vi "Ballard - Arinc-429 - Main Page.vi"(8 "error in (no error)":errorcluster, 11 "Node Ptr":T1 format="%.0x") -> (0 "error out":errorcluster)   [LabVIEW 2016, in "Ballard Arinc-429 System Explorer.lvlib"]
uses:
  Ballard Arinc-429 System Explorer.lvlib
  <vilib>/NI Veristand/Custom Device API/Custom Device Item Ref.ctl
  Shared/Controls and Global/Global.vi
  <vilib>/NI Veristand/Custom Device API/Get Item Property (Boolean).vi
  <vilib>/NI Veristand/Custom Device API/Get Item Property (Path).vi
  <vilib>/NI Veristand/Custom Device API/Get Item Property (String).vi
  <vilib>/NI Veristand/Custom Device API/Get Item Property (I32).vi
  <vilib>/NI Veristand/Custom Device API/Set Item Property (I32).vi
  <vilib>/NI Veristand/Custom Device API/Set Item Property (String).vi
  <vilib>/NI Veristand/Custom Device API/Custom Device API.lvlib
  Shared/Ballard Arinc-429 Shared.lvlib
  <vilib>/NI Veristand/Custom Device API/Set Item Property (Boolean).vi
panel:
  in  "Core Number":i32
  in  "Card Number":i32
  out "Version":string
  in  "ScheduledSDI?":bool
  in  "RefreshDB":bool
  in  "Warning text":string="WARNING: The database has changed since import. If you attempt to run this system definition an error may occur. Consider refreshing the database import."
  out "Warn Icon":bool
  out "Database File":path
  in  "Header":cluster{"Section Name":string}={"Section Name"="Ballard - Arinc-429 -  Custom Device"}
  in  "Description":string
  in  "Name":string
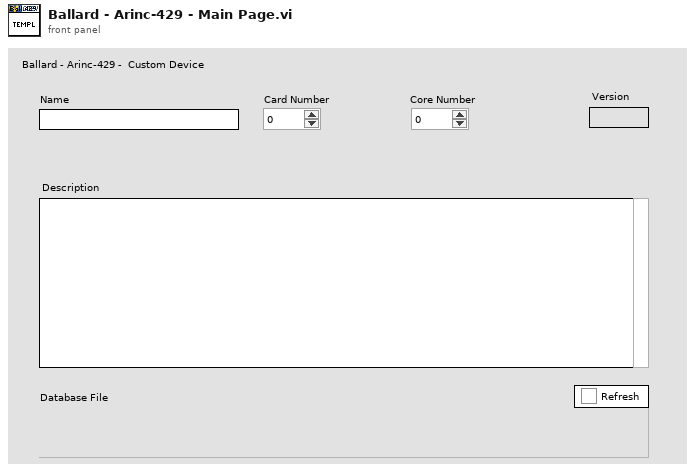
[diagram p1: front panel]
types:
  T1 = typedef "Custom Device API.lvlib/Custom Device Item Ref.ctl" = u64
  T2 = typedef "Custom Device API.lvlib/Custom Device Item Info.ctl" = cluster{"Name":string, "Is Channel":bool, "GUID":string, "Is Waveform":bool}
  T3 = typedef "Custom Device API.lvlib/Custom Device Commands.ctl" = enum16{"Default", "Item renamed", "Shutdown", "Dynamic button pressed"}
  T4 = typedef "Ballard Arinc-429 System Explorer.lvlib/Refresh Match Settings.ctl" = cluster{"Ch by name?":bool, "Lbl by name?":bool}
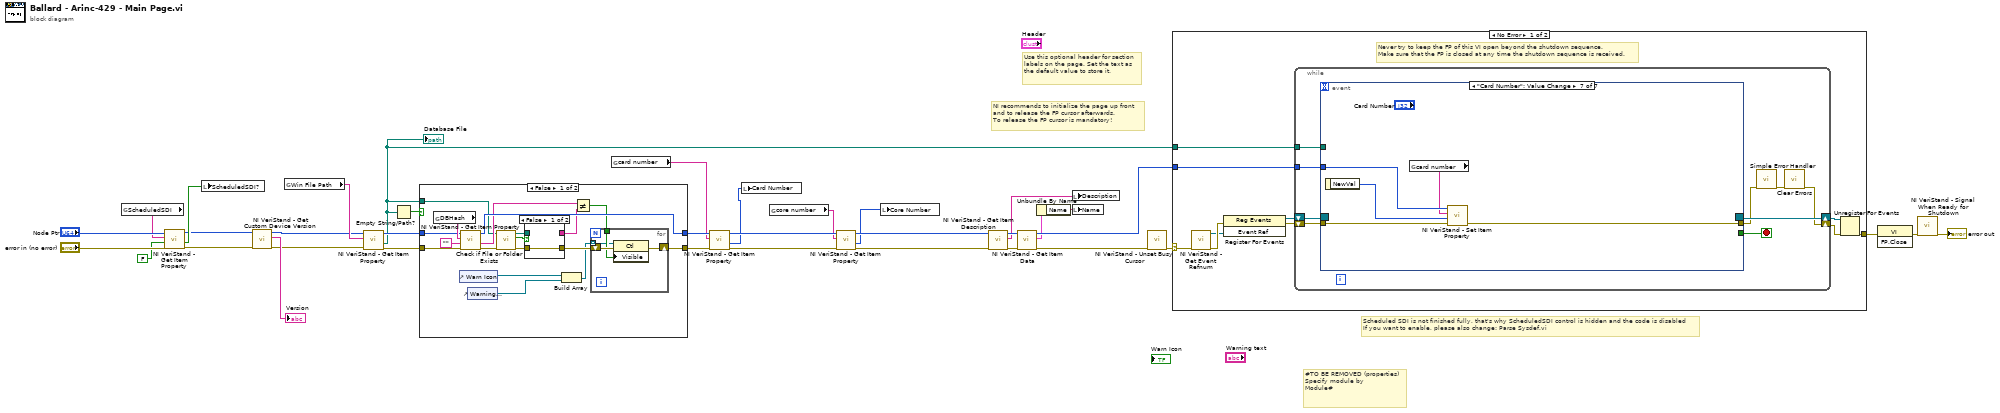
[diagram p0: block diagram]
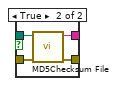
[diagram p2: hidden frame]
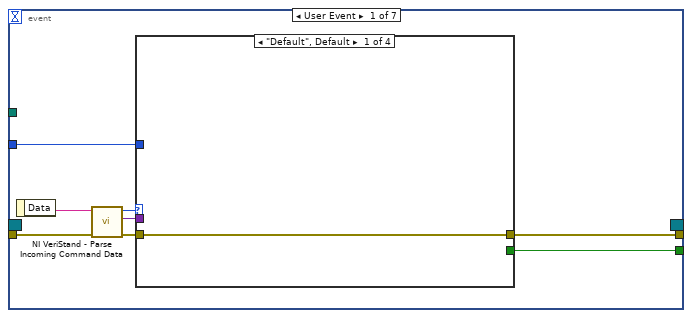
[diagram p4: hidden frame]
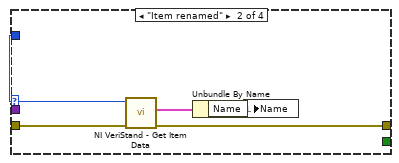
[diagram p5: hidden frame]
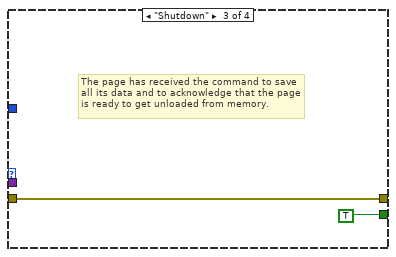
[diagram p6: hidden frame]
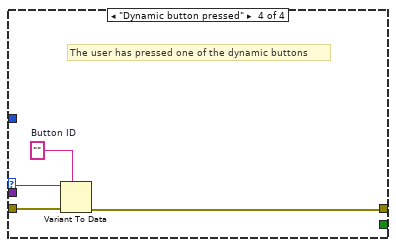
[diagram p7: hidden frame]
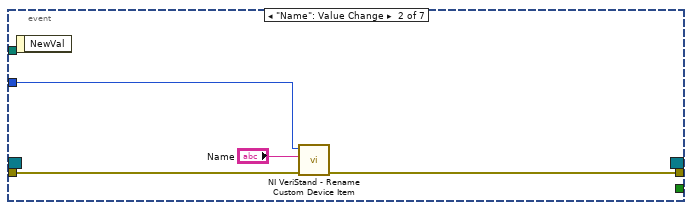
[diagram p8: hidden frame]
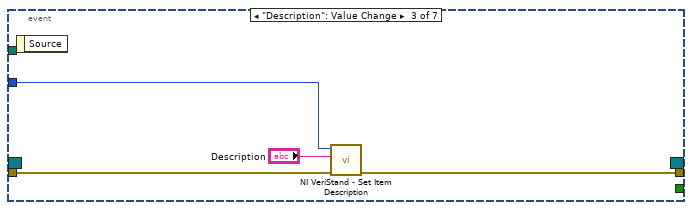
[diagram p9: hidden frame]
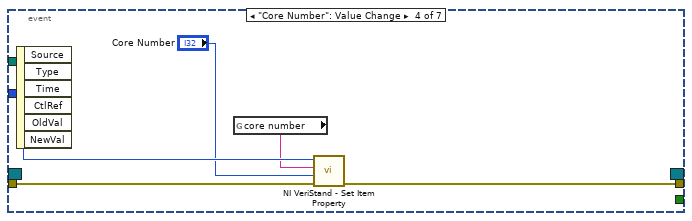
[diagram p10: hidden frame]
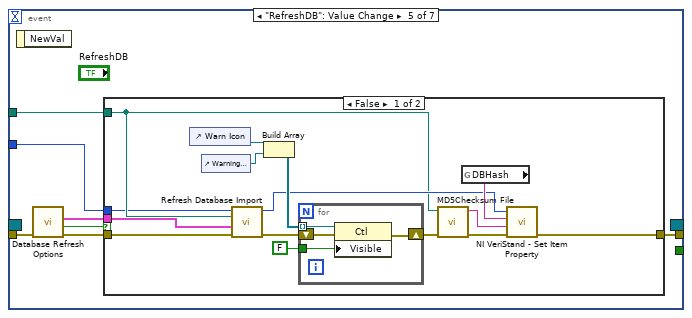
[diagram p11: hidden frame]
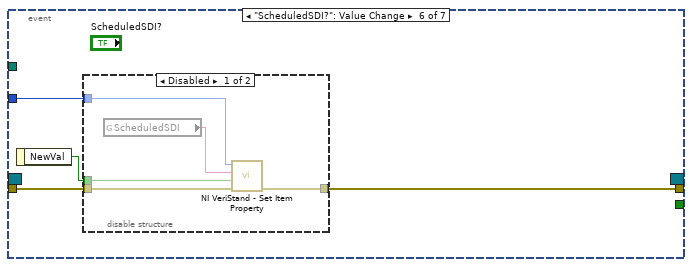
[diagram p13: hidden frame]
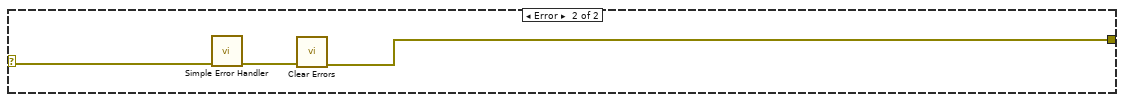
[diagram p15: hidden frame]
diagram:
  # "#TO BE REMOVED (properties)\nSpecify module by\nModule#"
  # "Scheduled SDI is not finished fully, that's why ScheduledSDI control is hidden and the code is disabled\nIf you want to enable, please also change: Parse Sysdef.vi"
  # "Use this optional header for section labels on the page. Set the text as the default value to store it."
  # "NI recommends to initialize the page up front\nand to release the FP cursor afterwards.\nTo release the FP cursor is mandatory!"
  n1 = global read "Global.vi" "ScheduledSDI"() -> (w15:string)
  n2 = call-poly <vilib>:"NI VeriStand - Get Item Property.vi"("error in (no error)"="error in (no error)", "Default Value"=FALSE, "Property Name"=w15, "Item Ref in"="Node Ptr") -> ("error out"=w16:errorcluster, "Value"=w13:bool, "Item Ref out"=w12:T1)  [unwired: 4 in, 1 out]
  n3 = local write "ScheduledSDI?"(w13) -> ()
  n4 = call <vilib>:"NI VeriStand - Get Custom Device Version.vi"("error in (no error)"=w16, "Device Ref in"=w12) -> ("error out"=w9:errorcluster, "Value"=→"Version":string, "Device Ref out"=w10:T1)  [unwired: 7 in]
  n5 = global read "Global.vi" "Win File Path"() -> (w25:string)
  n6 = call-poly <vilib>:"NI VeriStand - Get Item Property.vi"("error in (no error)"=w9, "Property Name"=w25, "Item Ref in"=w10) -> ("error out"=w23:errorcluster, "Value"=w19:path, "Item Ref out"=w20:T1)  [unwired: 5 in, 1 out]
  "Database File" <- w19
  n7 = Empty String/Path?(string/path=w19) -> (empty?=w24:bool)
  n8 = case shown="False" w24 {
    tunnel: w23 -> [w51 w65]
    tunnel: [w42 w65] -> w22
    tunnel: [w50 w64] -> w21
    tunnel: w20 -> [w52 w64]
    tunnel: w19 -> [w38 _]
    frame False {
      n9 = global read "Global.vi" "DBHash"() -> (w53:string)
      n10 = control-ref of="Warn Icon"() -> (w44:refnum<vi>)
      n11 = call-poly <vilib>:"NI VeriStand - Get Item Property.vi"("error in (no error)"=w51, "Default Value"="", "Property Name"=w53, "Item Ref in"=w52) -> ("error out"=w39:errorcluster, "Value"=w48:string, "Item Ref out"=w50:T1)  [unwired: 4 in, 1 out]
      n12 = control-ref of="Warning text"() -> (w45:refnum<vi>)
      n13 = call <vilib>:"Check if File or Folder Exists.vi"("error in (no error)"=w39, "path"=w38) -> ("error out"=w41:errorcluster, "file or folder exists?"=w37:bool, "dup path"=w40:path)  [unwired: 7 in]
      n14 = case shown="False" w37 {
        tunnel: [_ w59] -> w49
        tunnel: [w55 w58] -> w47
        tunnel: w41 -> [w55 w57]
        tunnel: w40 -> [_ w56]
        frame False {
        }
        frame True {
          n15 = call <vilib>:"MD5Checksum File.vi"("error in (no error)"=w57, "Path"=w56) -> ("error out"=w58:errorcluster, "MD5 message-digest"=w59:string)  [unwired: 8 in]
        }
      }
      n16 = Build Array(w44, w45) -> (w43:refnum<vi>[])
      n17 = Not Equal?(x=w48, y=w49) -> (x != y?=w46:bool)
      n18 = for {
        shift-right: [w62] -> w42
        shift-left: w47 -> [w63]
        tunnel: w46 -> [w61]
        tunnel: w43 -> [w60] mode=indexing
        n19 = property class="Ctl"(reference=w60, error in=w63, "Visible"=w61) -> (error out=w62:errorcluster)  [unwired: 1 out]
      }
    }
    frame True {
    }
  }
  n20 = global read "Global.vi" "card number"() -> (w2:string)
  n21 = call-poly <vilib>:"NI VeriStand - Get Item Property.vi"("error in (no error)"=w22, "Property Name"=w2, "Item Ref in"=w21) -> ("error out"=w5:errorcluster, "Value"=w1:i32, "Item Ref out"=w7:T1)  [unwired: 5 in, 1 out]
  n22 = local write "Card Number"(w1) -> ()
  n23 = global read "Global.vi" "core number"() -> (w3:string)
  n24 = call-poly <vilib>:"NI VeriStand - Get Item Property.vi"("error in (no error)"=w5, "Property Name"=w3, "Item Ref in"=w7) -> ("error out"=w8:errorcluster, "Value"=w4:i32, "Item Ref out"=w6:T1)  [unwired: 5 in, 1 out]
  n25 = local write "Core Number"(w4) -> ()
  n26 = call <vilib>:"NI VeriStand - Get Item Description.vi"("error in (no error)"=w8, "Item Ref in"=w6) -> ("error out"=w28:errorcluster, "Description"=w29:string, "Item Ref out"=w30:T1)  [unwired: 7 out]
  n27 = call <vilib>:"NI VeriStand - Get Item Data.vi"("error in (no error)"=w28, "Item Ref in"=w30) -> ("error out"=w33:errorcluster, "Item Info"=w27:T2, "Item Ref out"=w31:T1)  [unwired: 7 out]
  n28 = Unbundle By Name(w27) -> ("Name"=w26:string)
  n29 = local write "Description"(w29) -> ()
  n30 = local write "Name"(w26) -> ()
  n31 = call <vilib>:"NI VeriStand - Unset Busy Cursor.vi"("error in (no error)"=w33) -> ("error out"=w32:errorcluster)  [unwired: 10 out]
  n32 = case shown="No Error" w32 {
    selector: w32 -> [w67 w162]
    tunnel: [w72 w160] -> w36
    tunnel: w31 -> [w68 _]
    tunnel: w19 -> [w66 _]
    frame No Error {
      # "Never try to keep the FP of this VI open beyond the shutdown sequence.\nMake sure that the FP is closed at any time the shutdown sequence is received."
      n33 = call <vilib>:"NI VeriStand - Get Event Refnum.vi"("error in (no error)"=w67) -> ("error out"=w75:errorcluster, "Event Ref"=w71:refnum<user-event>)  [unwired: 9 out]
      n34 = register-events(error in=w75, w71) -> (reference out=w69:refnum<event-registration>, error out=w70:errorcluster)  [unwired: 1 in]
      n35 = while {
        tunnel: w68 -> [w80]
        shift-right: [w77] -> w73
        shift-left: w70 -> [w83]
        shift-right: [w84] -> w74
        shift-left: w69 -> [w82]
        tunnel: w66 -> [w76]
        stop <- w81 stop-if-true
        n36 = event shown="[6] \"Card Number\": Value Change" {
          selector: w82 -> [_ _ _ _ _ _ _]
          dyn-events: [_ _ _ _ _ _ _] -> w84
          timeout: _ -> [_ _ _ _ _ _ _]
          tunnel: w83 -> [w92 w108 w111 w117 w119 w148 w159]
          tunnel: [w88 _ _ _ _ _ _] -> w81
          tunnel: [w87 w107 w110 w116 w118 w145 w155] -> w79
          tunnel: w80 -> [w86 w106 w112 w115 w123 w147 w158]
          tunnel: w76 -> [_ _ _ _ w124 _ _]
          event User Event {
            n37 = event-data() -> ("Data"=w91:string)  [unwired: 1 out]
            n38 = call <vilib>:"NI VeriStand - Parse Incoming Command Data.vi"("error in (no error)"=w92, "Incoming data"=w91) -> ("error out"=w90:errorcluster, "Outgoing data"=w85:variant, "Action"=w89:T3)  [unwired: 7 out]
            n39 = case shown="\"Default\", Default" w89 {
              tunnel: w90 -> [w93 w98 w99 w104]
              tunnel: [_ _ TRUE _] -> w88
              tunnel: [w93 w95 w99 w101] -> w87
              tunnel: w86 -> [_ w97 _ _]
              tunnel: w85 -> [_ _ _ w103]
              frame "Default", Default {
              }
              frame "Item renamed" {
                n40 = call <vilib>:"NI VeriStand - Get Item Data.vi"("error in (no error)"=w98, "Item Ref in"=w97) -> ("error out"=w95:errorcluster, "Item Info"=w96:T2)  [unwired: 8 out]
                n41 = Unbundle By Name(w96) -> ("Name"=w94:string)
                n42 = local write "Name"(w94) -> ()
              }
              frame "Shutdown" {
                # "The page has received the command to save all its data and to acknowledge that the page is ready to get unloaded from memory."
              }
              frame "Dynamic button pressed" {
                w102 = ""  # Button ID
                # "The user has pressed one of the dynamic buttons"
                n43 = Variant To Data(error in=w104, type=w102, Variant=w103) -> (error out=w101:errorcluster)  [unwired: 1 out]
              }
            }
          }
          event "Name": Value Change {
            n44 = event-data() -> ()  [unwired: 2 out]
            n45 = call <vilib>:"NI VeriStand - Rename Custom Device Item.vi"("error in (no error)"=w108, "New Name"="Name", "Item Ref in"=w106) -> ("error out"=w107:errorcluster)  [unwired: 1 in, 7 out]
          }
          event "Description": Value Change {
            n46 = event-data() -> ()  [unwired: 2 out]
            n47 = call <vilib>:"NI VeriStand - Set Item Description.vi"("error in (no error)"=w111, "Description"="Description", "Item Ref in"=w112) -> ("error out"=w110:errorcluster)  [unwired: 8 out]
          }
          event "Core Number": Value Change {
            n48 = event-data() -> ()  [unwired: 7 out]
            n49 = global read "Global.vi" "core number"() -> (w113:string)
            n50 = call-poly <vilib>:"NI VeriStand - Set Item Property.vi"("error in (no error)"=w117, "Value"="Core Number", "Property Name"=w113, "Item Ref in"=w115) -> ("error out"=w116:errorcluster)  [unwired: 5 in, 2 out]
          }
          event "RefreshDB": Value Change {
            n51 = event-data() -> ()  [unwired: 2 out]
            n52 = call "Database Refresh Options.vi"("error in (no error)"=w119) -> ("error out"=w122:errorcluster, "Cancelled?"=w121:bool, "Refresh Settings"=w120:T4)  [unwired: 8 in]
            n53 = case shown="False" w121 {
              tunnel: [w126 w144] -> w118
              tunnel: w122 -> [w125 w144]
              tunnel: w124 -> [w129 _]
              tunnel: w123 -> [w128 _]
              tunnel: w120 -> [w127 _]
              frame False {
                n54 = control-ref of="Warn Icon"() -> (w135:refnum<vi>)
                n55 = control-ref of="Warning text"() -> (w136:refnum<vi>)
                n56 = call "Refresh Database Import.vi"("error in (no error)"=w125, "Match settings"=w127, "DB"=w129, "Item Ref in"=w128) -> ("error out"=w131:errorcluster, "Item Ref dup"=w130:T1)  [unwired: 5 in, 1 out]
                n57 = Build Array(w135, w136) -> (w133:refnum<vi>[])
                n58 = for {
                  shift-right: [w142] -> w134
                  shift-left: w131 -> [w143]
                  tunnel: w133 -> [w141] mode=indexing
                  tunnel: FALSE ("Visible") -> [w140]
                  n59 = property class="Ctl"(reference=w141, error in=w143, "Visible"=w140) -> (error out=w142:errorcluster)  [unwired: 1 out]
                }
                n60 = call <vilib>:"MD5Checksum File.vi"("error in (no error)"=w134, "Path"=w129) -> ("error out"=w139:errorcluster, "MD5 message-digest"=w138:string)  [unwired: 8 in]
                n61 = global read "Global.vi" "DBHash"() -> (w137:string)
                n62 = call-poly <vilib>:"NI VeriStand - Set Item Property.vi"("error in (no error)"=w139, "Value"=w138, "Property Name"=w137, "Item Ref in"=w130) -> ("error out"=w126:errorcluster)  [unwired: 5 in, 2 out]
              }
              frame True {
              }
            }
          }
          event "ScheduledSDI?": Value Change {
            n63 = event-data() -> ("NewVal"=w146:bool)  [unwired: 1 out]
            n64 = disable-structure shown="Disabled" {
              disable-tunnel: w148 -> [w153 w154]
              disable-tunnel: w147 -> [w152 _]
              disable-tunnel: w146 -> [w151 _]
              disable-tunnel: [w150 w154] -> w145
              frame Disabled {
                n65 = global read "Global.vi" "ScheduledSDI"() -> (w149:string)
                n66 = call-poly <vilib>:"NI VeriStand - Set Item Property.vi"("error in (no error)"=w153, "Value"=w151, "Property Name"=w149, "Item Ref in"=w152) -> ("error out"=w150:errorcluster)  [unwired: 5 in, 2 out]
              }
              frame Enabled {
              }
            }
          }
          event "Card Number": Value Change {
            n67 = event-data() -> ("NewVal"=w157:i32)  [unwired: 1 out]
            n68 = global read "Global.vi" "card number"() -> (w156:string)
            n69 = call-poly <vilib>:"NI VeriStand - Set Item Property.vi"("error in (no error)"=w159, "Value"=w157, "Property Name"=w156, "Item Ref in"=w158) -> ("error out"=w155:errorcluster)  [unwired: 5 in, 2 out]
          }
        }
        n70 = call <vilib>:"Simple Error Handler.vi"("error in (no error)"=w79) -> ("error out"=w78:errorcluster)  [unwired: 1 in, 7 out]
        n71 = call <vilib>:"Clear Errors.vi"("error in (no error)"=w78) -> ("error out"=w77:errorcluster)  [unwired: 1 in, 5 out]
      }
      n72 = Unregister For Events(event registration refnum=w74, error in=w73) -> (error out=w72:errorcluster)
    }
    frame Error {
      n73 = call <vilib>:"Simple Error Handler.vi"("error in (no error)"=w162) -> ("error out"=w161:errorcluster)  [unwired: 1 in, 7 out]
      n74 = call <vilib>:"Clear Errors.vi"("error in (no error)"=w161) -> ("error out"=w160:errorcluster)  [unwired: 1 in, 5 out]
    }
  }
  n75 = invoke class="VI" method="FP.Close"(error in=w36) -> (error out=w35:errorcluster)  [unwired: 2 in, 2 out]
  n76 = call <vilib>:"NI VeriStand - Signal When Ready for Shutdown.vi"("error in (no error)"=w35) -> ("error out"=→"error out":errorcluster)  [unwired: 10 out]
